vi "Test_Enumerate Service.vi"() -> ()   [LabVIEW 2020]
uses:
  Discovery_client/RPC Messages/NIMeasurementServices_EnumerateServicesRequest.ctl
  Discovery_client/RPC Messages/NIMeasurementServices_EnumerateServicesResponse.ctl
  Discovery_client/RPC Messages/NIMeasurementServices_ServiceDescriptor.ctl
  Discovery_client/Discovery_client.lvlib
panel:
  out "Response Data":T1
  in  "Request Data":T3
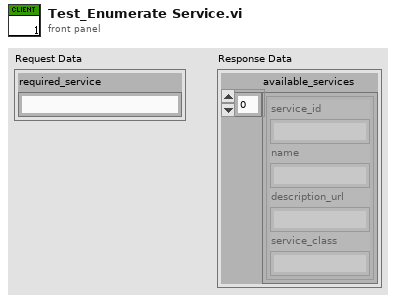
[diagram p1: front panel]
types:
  T1 = typedef "Discovery_client.lvlib/NIMeasurementServices_EnumerateServicesResponse.ctl" = cluster{"available_services":T2[]}
  T2 = typedef "Discovery_client.lvlib/NIMeasurementServices_ServiceDescriptor.ctl" = cluster{"service_id":string, "name":string, "description_url":string, "service_class":string}
  T3 = typedef "Discovery_client.lvlib/NIMeasurementServices_EnumerateServicesRequest.ctl" = cluster{"required_service":string}
  T4 = typedef "gprc-lvsupport-release.lvlib/grpcId.ctl" = u64
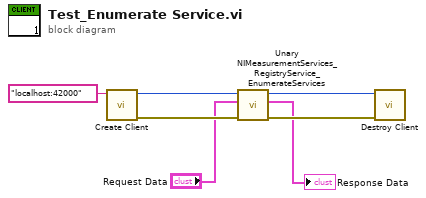
[diagram p0: block diagram]
diagram:
  n1 = call "Create Client.vi"("address"="localhost:42000") -> ("error out"=w5:errorcluster, "gRPC ID Out"=w6:T4)  [unwired: 9 in]
  n2 = call "Unary NIMeasurementServices_RegistryService_EnumerateServices.vi"("error in"=w5, "Request Data"="Request Data", "gRPC ID"=w6) -> ("error out"=w4:errorcluster, "Response Data"=→"Response Data":T1, "gRPC ID out"=w3:T4)  [unwired: 6 in]
  n3 = call "Destroy Client.vi"("error in"=w4, "gRPC ID"=w3) -> ()  [unwired: 9 in, 1 out]
